vi "CubeLiftAuto.vi"() -> ()   [LabVIEW 2017]
uses:
  AutoSubsystem/AutoOutput.ctl
  AutoSubsystem/AutoSubroutine.lvclass
  AutoSubsystem/AutoInput.ctl
panel:
  out "AutoGeneralOut":T1
  in  "GeneralAutoInput":T2
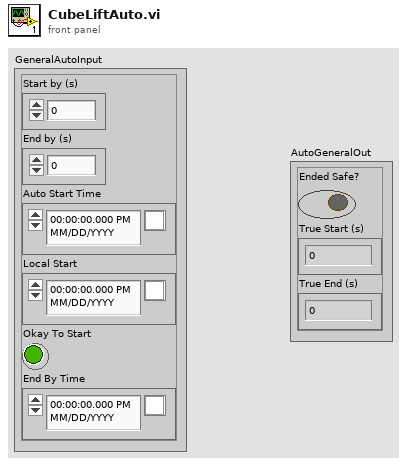
[diagram p1: front panel]
types:
  T1 = typedef "AutoSubroutine.lvclass/AutoOutput.ctl" = cluster{"Ended Safe?":bool, "True Start (s)":dbl, "True End (s)":dbl}
  T2 = typedef "AutoSubroutine.lvclass/AutoInput.ctl" = cluster{"Start by (s)":dbl, "End by (s)":dbl, "Auto Start Time":timestamp, "Local Start":timestamp, "Okay To Start":bool, "End By Time":timestamp}
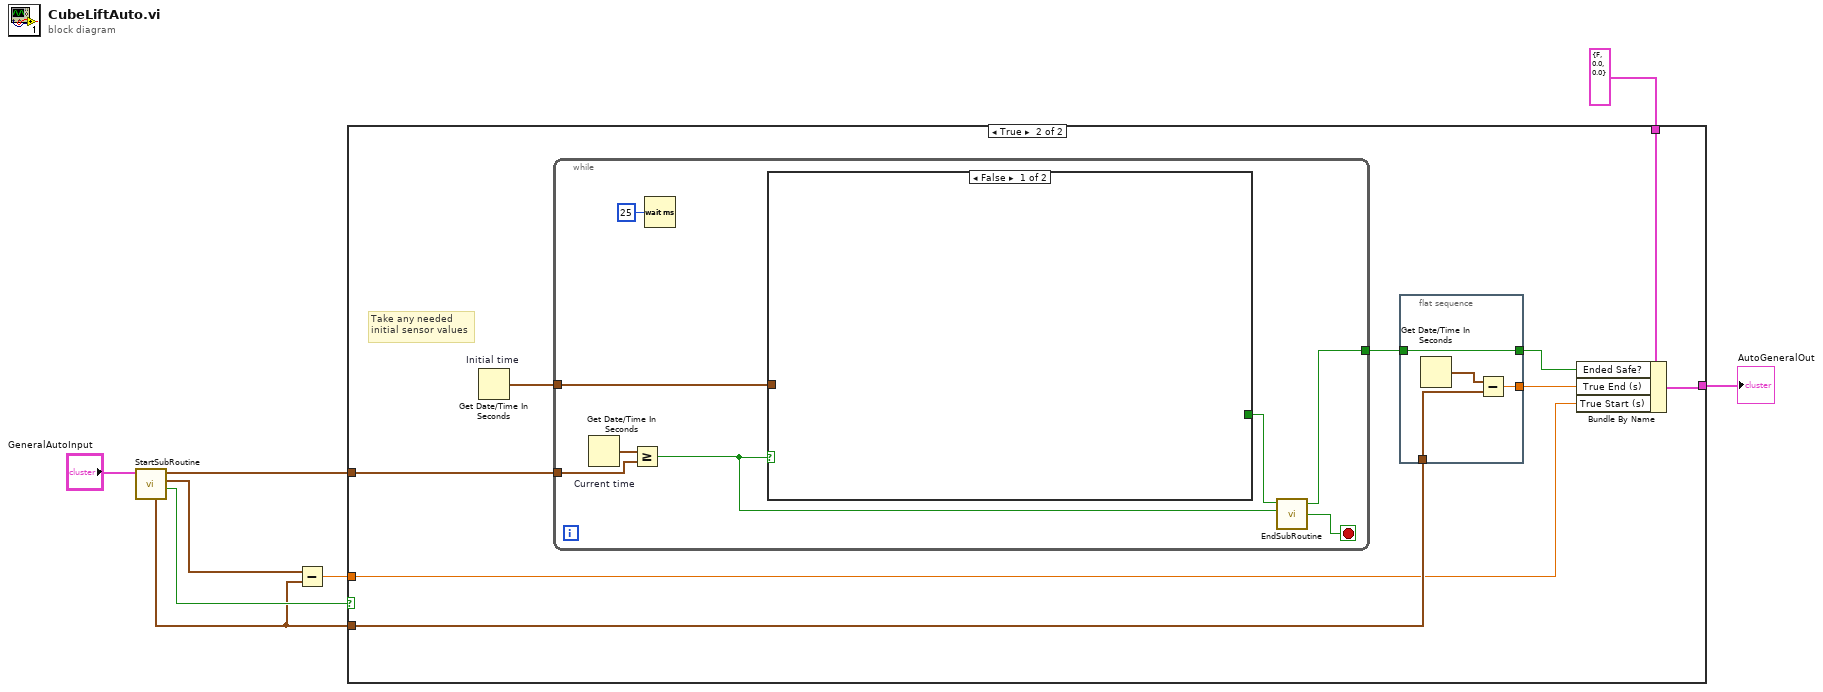
[diagram p0: block diagram]
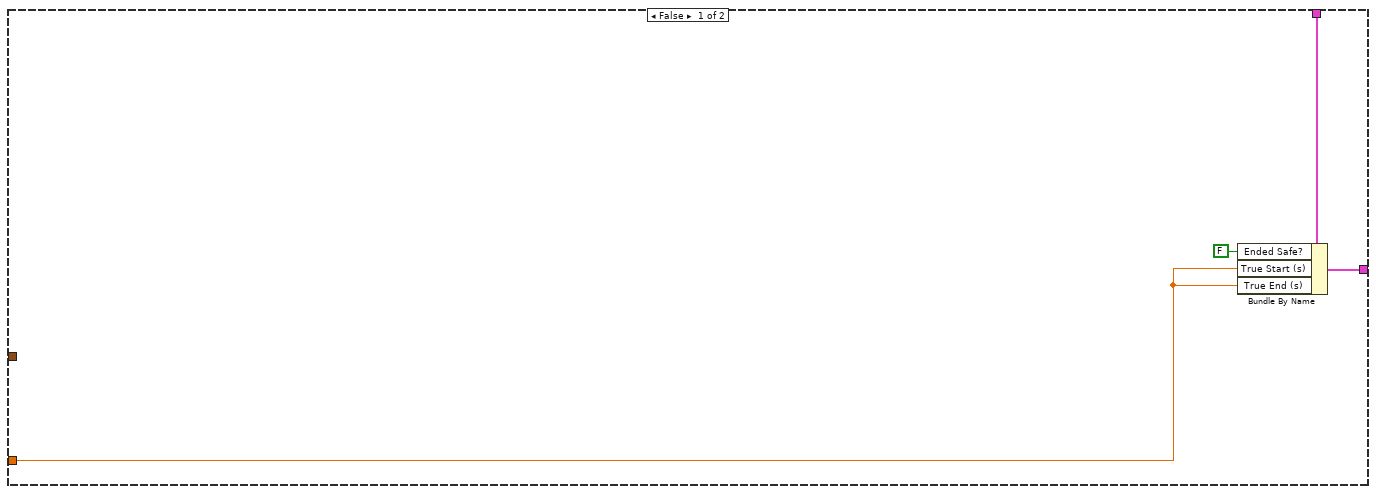
[diagram p2: hidden frame]
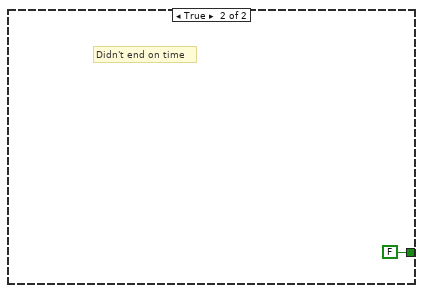
[diagram p3: hidden frame]
diagram:
  n1 = call "StartSubRoutine.vi"("GeneralAutoInput"="GeneralAutoInput") -> ("Okay to start?"=w4:bool, "Local Start"=w3:timestamp, "End by:"=w5:timestamp, "Auto Start Time"=w2:timestamp)  [unwired: 7 in]
  n2 = Subtract(x=w3, y=w2) -> (x-y=w1:dbl)
  n3 = case shown="True" w4 {
    tunnel: [w11 w19] -> w8
    tunnel: w5 -> [_ w21]
    tunnel: T1 {"Ended Safe?"=FALSE, "True Start (s)"=0.0, "True End (s)"=0.0} ("AutoGeneralOut 2") -> [w12 w20]
    tunnel: w2 -> [_ w18]
    tunnel: w1 -> [w9 w17]
    frame False {
      n4 = Bundle By Name(cluster=w12, "Ended Safe?"=FALSE, "True Start (s)"=w9, "True End (s)"=w9) -> (w11:T1)
    }
    frame True {
      # "Take any needed\ninitial sensor values"
      n5 = Get Date/Time In Seconds "Initial time"() -> (seconds since 1Jan1904=w13:timestamp)
      n6 = while {
        tunnel: w21 -> [w32]
        tunnel: [w29] -> w14
        tunnel: w13 -> [w27]
        stop <- w30 stop-if-true
        n7 = Get Date/Time In Seconds "Current time"() -> (seconds since 1Jan1904=w33:timestamp)
        n8 = Greater Or Equal?(x=w33, y=w32) -> (x >= y?=w26:bool)
        n9 = Wait (ms)(milliseconds to wait=u32 25) -> ()  [unwired: 1 out]
        n10 = case shown="False" w26 {
          tunnel: [_ FALSE ("Done?")] -> w31
          tunnel: w27 -> [_ _]
          frame False {
          }
          frame True {
            # "Didn't end on time"
          }
        }
        n11 = call "EndSubRoutine.vi"("Done?"=w31, "Ran too long?"=w26) -> ("Safe Stop?"=w29:bool, "Stop?"=w30:bool)  [unwired: 5 in]
      }
      n12 = flat-sequence {
        tunnel: w18 -> [w24]
        tunnel: [w23] -> w16
        tunnel: [w22] -> w15
        tunnel: w14 -> [w22]
        frame #0 {
          n13 = Get Date/Time In Seconds() -> (seconds since 1Jan1904=w25:timestamp)
          n14 = Subtract(x=w25, y=w24) -> (x-y=w23:dbl)
        }
      }
      n15 = Bundle By Name(cluster=w20, "Ended Safe?"=w15, "True End (s)"=w16, "True Start (s)"=w17) -> (w19:T1)
    }
  }
  "AutoGeneralOut" <- w8
